vi "Get Moving Status.vi"(8 "error in (no error)":errorcluster, 11 "Axis in":refnum<class "Axis.lvclass">) -> (0 "error out":errorcluster, 2 "Moving?":bool, 3 "Axis out":refnum<class "Axis.lvclass">)   [LabVIEW 2018, in "Axis.lvlib" / "Axis.lvclass"]
uses:
  Axis.lvclass
  Custom Controls/Command.ctl
  Axis.lvclass/Axis.ctl
  Axis.lvlib
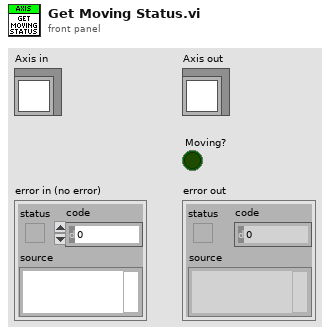
[diagram p1: front panel]
types:
  T1 = typedef "Axis.lvlib/Command.ctl" = enum16{"None", "Home", "Renumber", "Move Absolute", "Move Relative", "Stop", "Set Run Speed", "Set Acceleration", "Set Run Current", "Set Home Offset", "Set Home Speed", "Query Current Position", "Load Defaults", "Query Status", "Lock Controls", "Unlock Controls", "Set Jog Step Size", "Set Jog Acceleration", "Set Jog Speed", "Query Homed Status", "Query Moving Status", "Reset", "Set Max Position", "Set Min Position"}
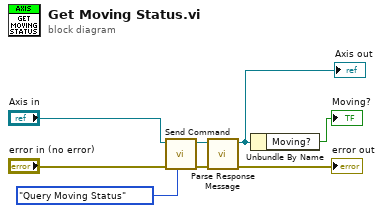
[diagram p0: block diagram]
diagram:
  n1 = call-dynamic "Send Command.vi"("Command"=Command."Query Moving Status", "error in"="error in (no error)", "Axis in"="Axis in") -> ("error out"=w6:errorcluster, "Axis out"=w7:refnum<class "Axis.lvclass">)  [unwired: 7 in]
  n2 = call-dynamic "Parse Response Message.vi"("error in"=w6, "Axis in"=w7) -> ("error out"=→"error out":errorcluster, "Axis out"=w2:refnum<class "Axis.lvclass">)  [unwired: 8 in]
  "Axis out" <- w2
  n3 = Unbundle By Name(w2) -> ("Moving?"=→"Moving?":bool)
